vi "Configure Control Mode.vi"(8 "error in (no error)":errorcluster, 10 "control mode":u16(ring)=1 items=["manual"=1, "analog"=2, "auto"=3], 11 "MKS MW in":refnum<class "PL MKS MW.lvclass">) -> (0 "error out":errorcluster, 3 "MKS MW out":refnum<class "PL MKS MW.lvclass">)   [LabVIEW 2015, in "PL MKS MW.lvclass"]
doc: "Configures device control mode (manual/auto/analog)."
uses:
  PL MKS MW.lvclass
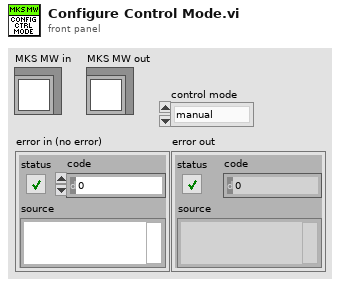
[diagram p1: front panel]
types:
  T1 = cluster{"Udc, V":u16, "Upp, V":u16, "C1, %":u8, "C2, %":u8, "control mode":u16, "preset":u16}
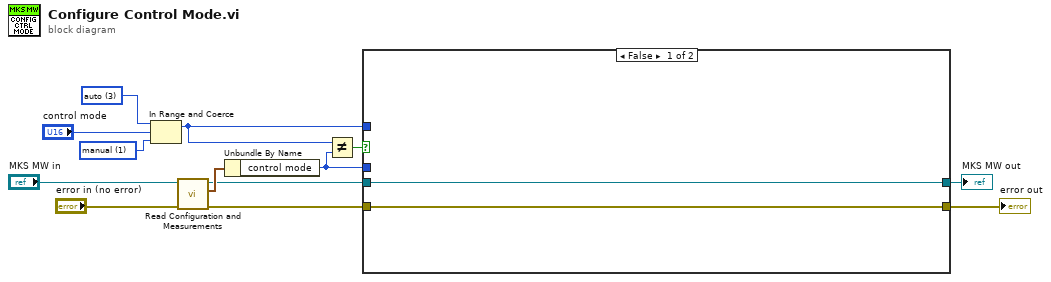
[diagram p0: block diagram]
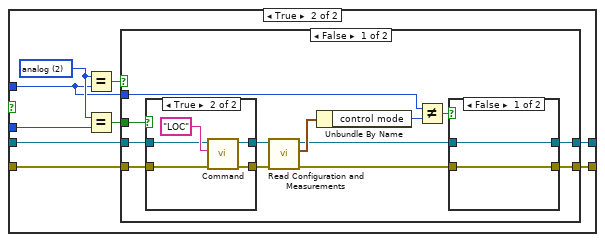
[diagram p2: hidden frame]
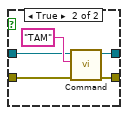
[diagram p3: hidden frame]
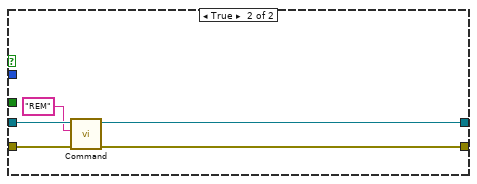
[diagram p5: hidden frame]
diagram:
  w11 = u16 3 items=["manual"=1, "analog"=2, "auto"=3] ("control mode")
  w12 = u16 1 items=["manual"=1, "analog"=2, "auto"=3] ("control mode")
  n1 = In Range and Coerce(upper limit=w11, x="control mode", lower limit=w12) -> (coerced(x)=w2:u16)  [unwired: 1 out]
  n2 = call "Read Configuration and Measurements.vi"("error in (no error)"="error in (no error)", "MKS MW in"="MKS MW in") -> ("error out"=w4:errorcluster, "configuration and measurements"=w8:T1, "MKS MW out"=w7:refnum<class "PL MKS MW.lvclass">)  [unwired: 7 in]
  n3 = Unbundle By Name(w8) -> ("control mode"=w1:u16)
  n4 = Not Equal?(x=w2, y=w1) -> (x != y?=w6:bool)
  n5 = case shown="False" w6 {
    tunnel: w7 -> [w15 w24]
    tunnel: [w15 w22] -> w5
    tunnel: w4 -> [w14 w23]
    tunnel: [w14 w21] -> w3
    tunnel: w2 -> [_ w16]
    tunnel: w1 -> [_ w18]
    frame False {
    }
    frame True {
      w19 = u16 2 items=["manual"=1, "analog"=2, "auto"=3] ("control mode")
      n6 = Equal?(x=w19, y=w16) -> (x = y?=w20:bool)
      n7 = Equal?(x=w19, y=w18) -> (x = y?=w17:bool)
      n8 = case shown="False" w20 {
        tunnel: w24 -> [w36 w56]
        tunnel: w23 -> [w35 w55]
        tunnel: [w26 w54] -> w22
        tunnel: [w25 w53] -> w21
        tunnel: w17 -> [w37 _]
        tunnel: w16 -> [w30 _]
        frame False {
          n9 = case shown="True" w37 {
            tunnel: w36 -> [w46 w50]
            tunnel: w35 -> [w45 w49]
            tunnel: [w46 w48] -> w34
            tunnel: [w45 w47] -> w33
            frame False {
            }
            frame True {
              n10 = call "Command.vi"("error in (no error)"=w49, "command"="LOC", "MKS MW in"=w50) -> ("error out"=w47:errorcluster, "MKS MW out"=w48:refnum<class "PL MKS MW.lvclass">)  [unwired: 6 in, 1 out]
            }
          }
          n11 = call "Read Configuration and Measurements.vi"("error in (no error)"=w33, "MKS MW in"=w34) -> ("error out"=w27:errorcluster, "configuration and measurements"=w32:T1, "MKS MW out"=w28:refnum<class "PL MKS MW.lvclass">)  [unwired: 7 in]
          n12 = Unbundle By Name(w32) -> ("control mode"=w31:u16)
          n13 = Not Equal?(x=w30, y=w31) -> (x != y?=w29:bool)
          n14 = case shown="False" w29 {
            tunnel: w28 -> [w39 w43]
            tunnel: w27 -> [w38 w42]
            tunnel: [w39 w41] -> w26
            tunnel: [w38 w40] -> w25
            frame False {
            }
            frame True {
              n15 = call "Command.vi"("error in (no error)"=w42, "command"="TAM", "MKS MW in"=w43) -> ("error out"=w40:errorcluster, "MKS MW out"=w41:refnum<class "PL MKS MW.lvclass">)  [unwired: 6 in, 1 out]
            }
          }
        }
        frame True {
          n16 = call "Command.vi"("error in (no error)"=w55, "command"="REM", "MKS MW in"=w56) -> ("error out"=w53:errorcluster, "MKS MW out"=w54:refnum<class "PL MKS MW.lvclass">)  [unwired: 6 in, 1 out]
        }
      }
    }
  }
  "MKS MW out" <- w5
  "error out" <- w3
